vi "QTrkComputeZLUTBiasTable.vi"(6 "Use spline interpolation?":bool, 8 "error in (no error)":errorcluster, 9 "smpPerPixel":i32=4, 10 "bias planes":i32, 11 "QTrk Instance":T1) -> (0 "error out":errorcluster, 1 "Bias correction table":sgl[][](array[numeric]), 3 "QTrk Instance":T1)   [LabVIEW 2011]
uses:
  QTrkInstance.ctl
  QTrkDLL.vi
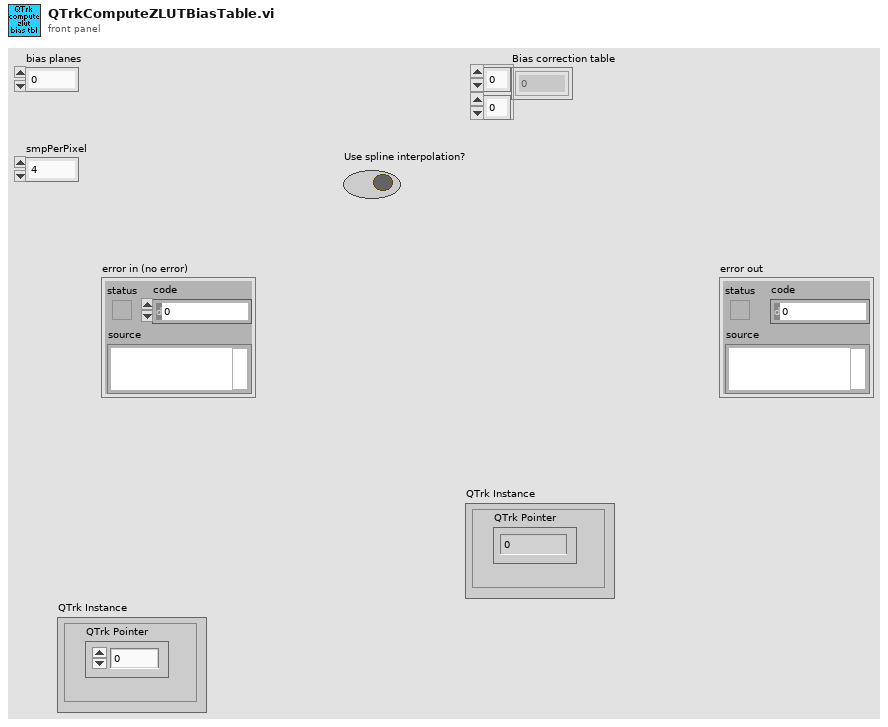
[diagram p1: front panel]
types:
  T1 = typedef "QTrkInstance.ctl" = cluster{"QTrk Pointer":u64}
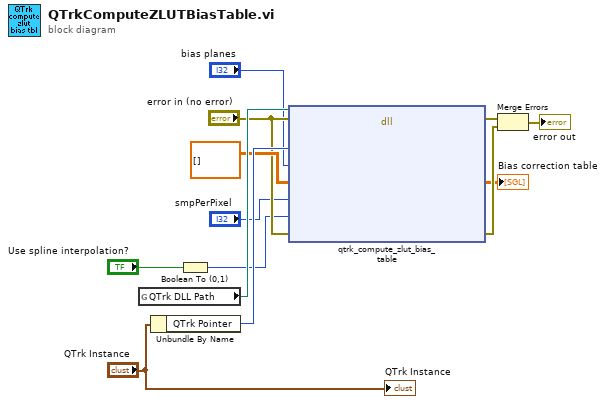
[diagram p0: block diagram]
diagram:
  n1 = global read "QTrkDLL.vi" "QTrk DLL Path"() -> (w11:path)
  n2 = Unbundle By Name("QTrk Instance") -> ("QTrk Pointer"=w12:u64)
  n3 = Boolean To (0,1)(Boolean="Use spline interpolation?") -> (0, 1=w1:i16)
  n4 = dll-call lib="D:/jcnossen1/cudaqi-tracker/bin/jtrk-labview.dll" fn="qtrk_compute_zlut_bias_table"(path in=w11, error in="error in (no error)", "tracker"=w12, "bias planes"="bias planes", "result"=sgl[][] [] ("Bias correction table"), "smpPerPixel"="smpPerPixel", "useSplineInterp"=w1, "error in (no error)") -> (error out=w9:errorcluster, "result"=→"Bias correction table":sgl[][], w10:errorcluster)  [unwired: 6 in, 1 out]
  n5 = Merge Errors(w9, w10) -> (→"error out":errorcluster)
  "QTrk Instance" <- "QTrk Instance"
